vi "Baretail.vi"(8 "error in (no error)":errorcluster, 10 "PATH":path) -> (0 "error out":errorcluster, 2 "path":path)   [LabVIEW 2018]
panel:
  out "standard output":string
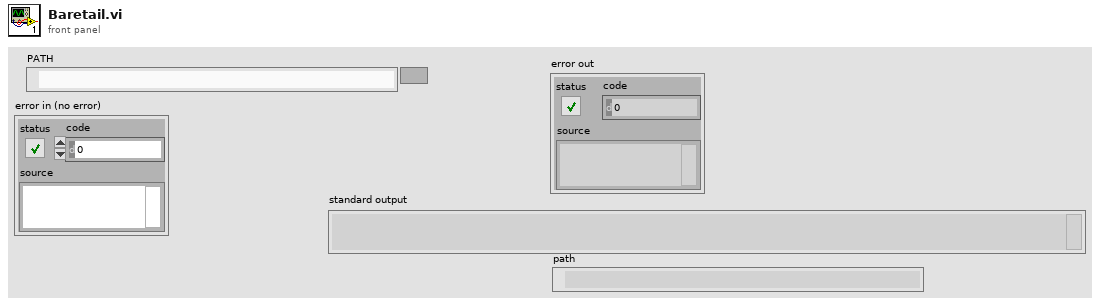
[diagram p1: front panel]
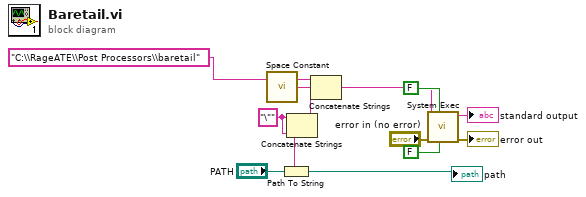
[diagram p0: block diagram]
diagram:
  w1 = "\"" ("string")
  n1 = call <vilib>:"Space Constant.vi"() -> ("String"=w8:string)
  n2 = Path To String(path="PATH") -> (string=w7:string)
  n3 = Concatenate Strings(w1, w7, w1) -> (w2:string)
  n4 = Concatenate Strings("C:\\RageATE\\Post Processors\\baretail" ("command line"), w8, w2) -> (w9:string)
  n5 = call <vilib>:"System Exec.vi"("run minimized? (F)"=FALSE, "wait until completion? (T)"=FALSE, "error in (no error)"="error in (no error)", "command line"=w9) -> ("error out"=→"error out":errorcluster, "standard output"=→"standard output":string)  [unwired: 4 in, 2 out]
  "path" <- "PATH"
